vi "Test MQTT-3.3.2-2.vi"(8 "error in (no error)":errorcluster) -> (0 "error out":errorcluster)   [LabVIEW 2013]
uses:
  <vilib>/addons/_JKI Toolkits/Caraya/classes/Test/Test.lvclass
  source/Control Packets/PUBLISH/PUBLISH.lvclass
  <vilib>/addons/_JKI Toolkits/Caraya/classes/Assert/Assert.lvclass
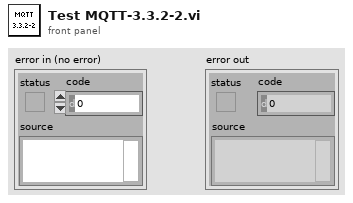
[diagram p1: front panel]
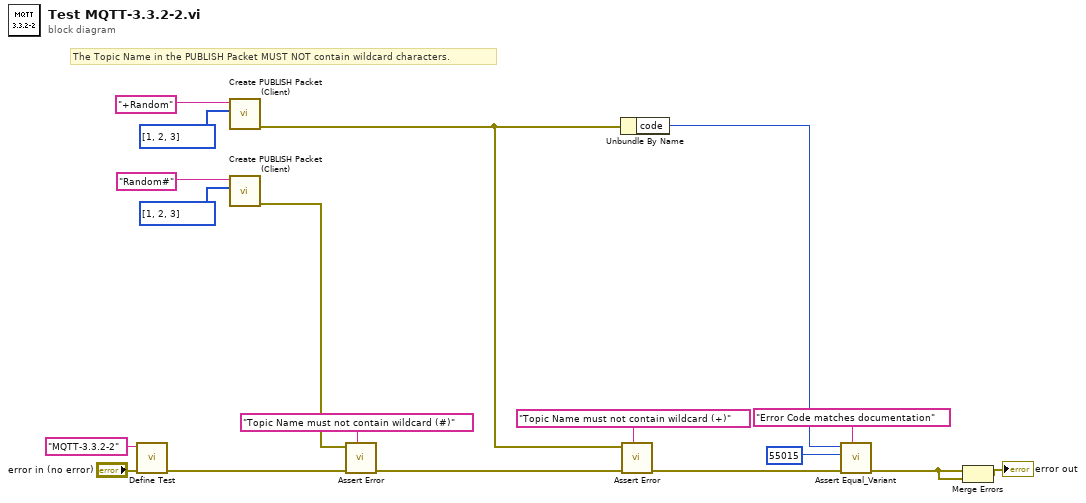
[diagram p0: block diagram]
diagram:
  # "The Topic Name in the PUBLISH Packet MUST NOT contain wildcard characters."
  n1 = call <vilib>:"Define Test.vi"("error in (no error)"="error in (no error)", "Label (VI Title)"="MQTT-3.3.2-2") -> ("error out"=w15:errorcluster)  [unwired: 9 in]
  n2 = call "Create PUBLISH Packet (Client).vi"("Payload"=u8[] [1, 2, 3], "Topic Name"="+Random" ("Client ID (empty: generate new)")) -> ("error out"=w6:errorcluster)  [unwired: 7 in, 2 out]
  n3 = call "Create PUBLISH Packet (Client).vi"("Payload"=u8[] [1, 2, 3], "Topic Name"="Random#" ("Client ID (empty: generate new)")) -> ("error out"=w9:errorcluster)  [unwired: 7 in, 2 out]
  n4 = call <vilib>:"Assert Error.vi"("Label"="Topic Name must not contain wildcard (#)", "error in (no error)"=w15, "Error?"=w9) -> ("error out"=w10:errorcluster)  [unwired: 8 in]
  n5 = Unbundle By Name(w6) -> ("code"=w4:i32)
  n6 = call <vilib>:"Assert Error.vi"("Label"="Topic Name must not contain wildcard (+)", "error in (no error)"=w10, "Error?"=w6) -> ("error out"=w2:errorcluster)  [unwired: 8 in]
  n7 = call <vilib>:"Assert Equal_Variant.vi"("Label"="Error Code matches documentation", "error in (no error)"=w2, "Y"=55015 ("code"), "X"=w4) -> ("error out"=w1:errorcluster)  [unwired: 7 in]
  n8 = Merge Errors(w1, w1) -> (→"error out":errorcluster)
